vi "Read Variable (boolean).vi"(8 "error in (no error)":errorcluster, 9 "Datatype":bool, 10 "PG path":string, 11 "Data.PGQL in":refnum<class "LV-Data.PGSQL.lvclass">) -> (0 "error out":errorcluster, 1 "Time Stamp":timestamp, 2 "Value":bool, 3 "Data.PGSQL out":refnum<class "LV-Data.PGSQL.lvclass">, 4 "Column (units)":string, 5 "SQL string":string)   [LabVIEW 2019, in "LV-Data.PGSQL.lvclass"]
uses:
  LV-Data.PGSQL.lvclass
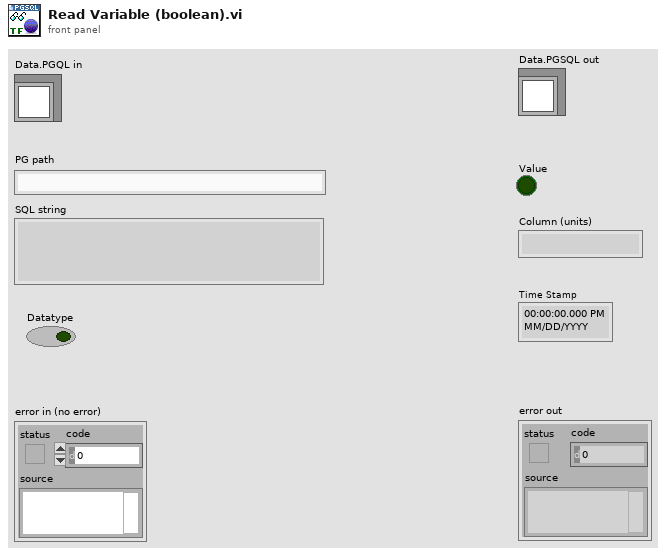
[diagram p1: front panel]
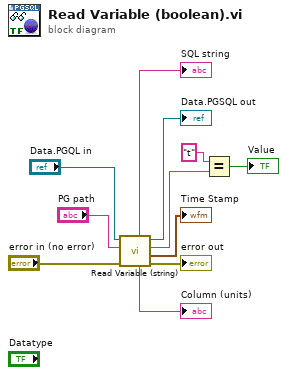
[diagram p0: block diagram]
diagram:
  n1 = call "Read Variable (string).vi"("error in (no error)"="error in (no error)", "PG path"="PG path", "Data.PGQL in"="Data.PGQL in") -> ("error out"=→"error out":errorcluster, "Time Stamp"=→"Time Stamp":timestamp, "Value"=w9:string, "Data.PGSQL out"=→"Data.PGSQL out":refnum<class "LV-Data.PGSQL.lvclass">, "Column (units)"=→"Column (units)":string, "SQL string"=→"SQL string":string)  [unwired: 3 in]
  n2 = Equal?(x="t", y=w9) -> (x = y?=→"Value":bool)
